vi "Compare Versions.vi"(8 "error in (no error)":errorcluster, 10 "Version 2":string, 11 "Version 1":string) -> (0 "error out":errorcluster, 1 "Version 1 Lesser?":bool, 2 "Equal?":bool, 3 "Version 1 Greater?":bool)   [LabVIEW 2016, in "SLL Application.lvlib"]
doc: "Compares two versions and returns whether the version 1 is greater, or equal to, or lesser than what is specified for version 2.\n\nThe number of digits in the version number can also vary which is also handled. Eg:\nVersion 1: 1.0.\nVersion 2: 1.0.0.1"
uses:
  SLL Application.lvlib
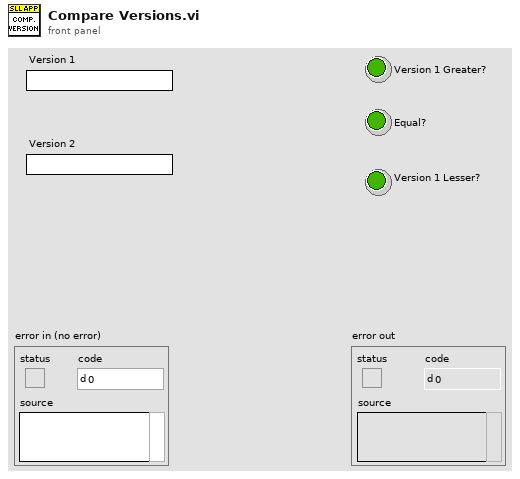
[diagram p1: front panel]
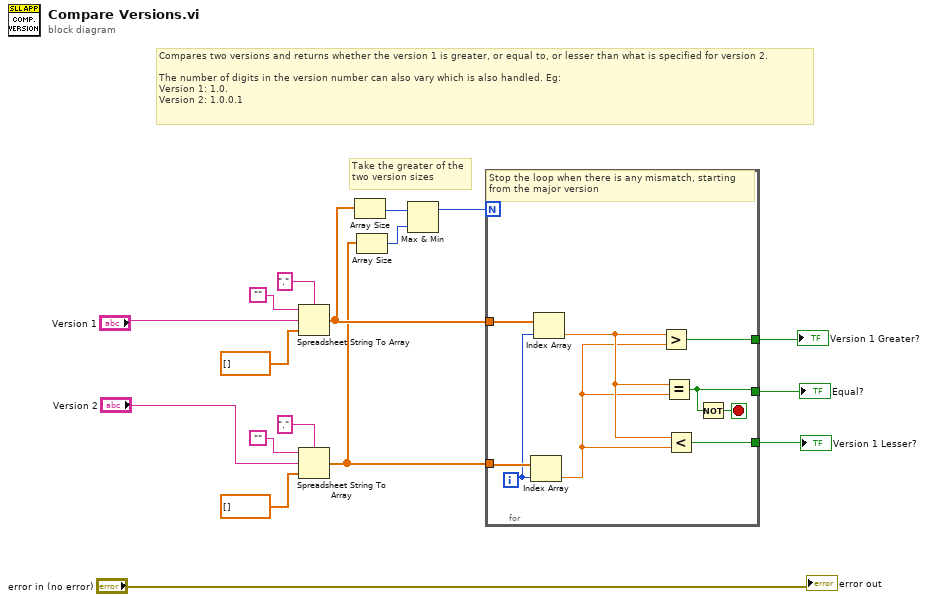
[diagram p0: block diagram]
diagram:
  # "Compares two versions and returns whether the version 1 is greater, or equal to, or lesser than what is specified for version 2.\n\nThe number of digits in the version number can also vary which is also handled. Eg:\nVersion 1: 1.0.\nVersion 2: 1.0.0.1"
  # "Take the greater of the\ntwo version sizes"
  n1 = Spreadsheet String To Array(delimiter (Tab)=".", format string="", spreadsheet string="Version 1", array type (2D Dbl)=dbl[] []) -> (array=w6:dbl[])
  n2 = Spreadsheet String To Array(delimiter (Tab)=".", format string="", spreadsheet string="Version 2", array type (2D Dbl)=dbl[] []) -> (array=w5:dbl[])
  n3 = Array Size(array=w6) -> (size(s)=w9:i32)
  n4 = Array Size(array=w5) -> (size(s)=w8:i32)
  n5 = Max & Min(x=w9, y=w8) -> (max(x,y)=w7:i32)  [unwired: 1 out]
  n6 = for {
    N: w7 -> [_]
    tunnel: w6 -> [w26]
    tunnel: w5 -> [w25]
    tunnel: [w20] -> w4
    tunnel: [w19] -> w2
    tunnel: [w18] -> w3
    i -> [w24]
    stop <- w21 stop-if-true
    # "Stop the loop when there is any mismatch, starting from the major version"
    n7 = Index Array(array=w25, index=w24) -> (element=w22:dbl)
    n8 = Index Array(array=w26, index=w24) -> (element=w23:dbl)
    n9 = Greater?(x=w23, y=w22) -> (0:w20:bool)
    n10 = Equal?(x=w23, y=w22) -> (x = y?=w18:bool)
    n11 = Less?(x=w23, y=w22) -> (x < y?=w19:bool)
    n12 = Not(x=w18) -> (.not. x?=w21:bool)
  }
  "Version 1 Greater?" <- w4
  "Equal?" <- w3
  "Version 1 Lesser?" <- w2
  "error out" <- "error in (no error)"
